vi "Save data file (pass-fail) & report v1.vi"(8 "Input Cluster":T1, 11 "panel id":string) -> (0 "network file save error":errorcluster, 3 "file save path":string)   [LabVIEW 2013]
uses:
  program files/Global 1.vi
  program files/Global display 2.vi
  program files/Global display 3.vi
  <vilib>/Utility/NIReport.llb/NI_report.lvclass
panel:
  out "status":string
  out "C drive root path":string
  out "network file dir path":path
  out "network dir":string
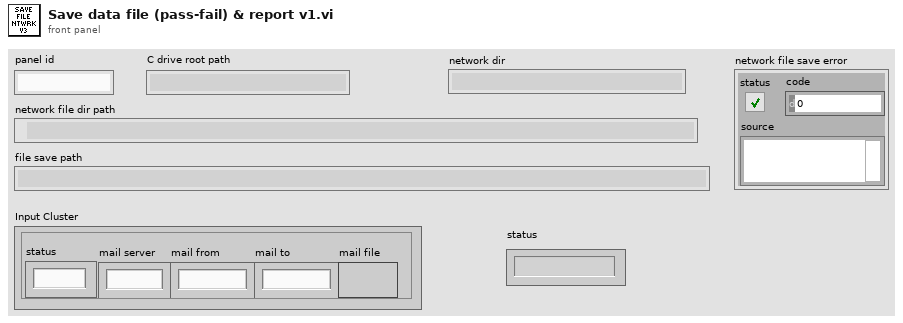
[diagram p1: front panel]
types:
  T1 = cluster{"status":string, "mail server":string, "mail from":string, "mail to":string, "mail file":bool}
  T2 = cluster{"CYCLE":dbl, "MINS":dbl, "STATUS":string}
  T3 = cluster{"NAME":string, "DESCRIPTION":string, "CYCLES":dbl, "T-RISE mins":dbl, "T-RISE deg C":dbl}
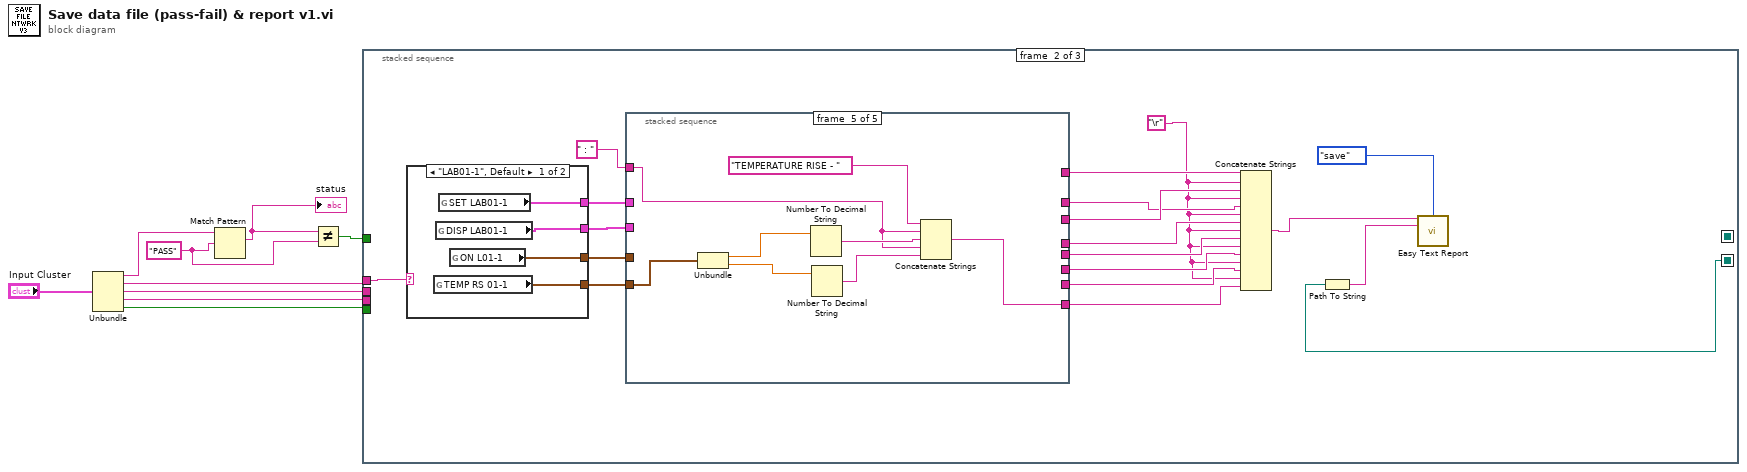
[diagram p0: block diagram]
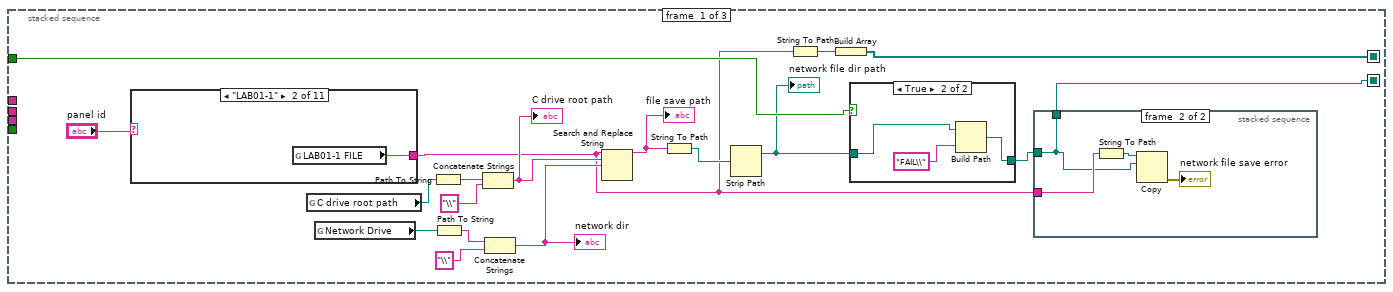
[diagram p2: hidden frame]
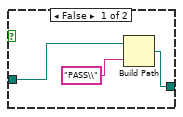
[diagram p3: hidden frame]
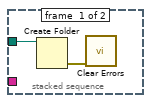
[diagram p4: hidden frame]
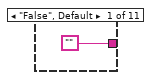
[diagram p5: hidden frame]
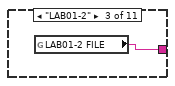
[diagram p6: hidden frame]
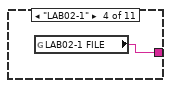
[diagram p7: hidden frame]
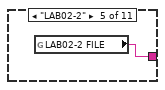
[diagram p8: hidden frame]
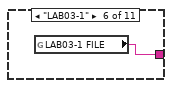
[diagram p9: hidden frame]
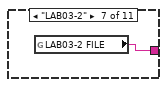
[diagram p10: hidden frame]
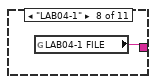
[diagram p11: hidden frame]
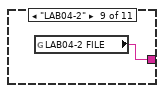
[diagram p12: hidden frame]
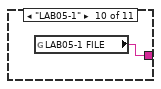
[diagram p13: hidden frame]
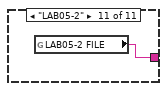
[diagram p14: hidden frame]
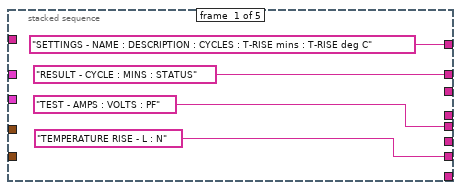
[diagram p15: hidden frame]
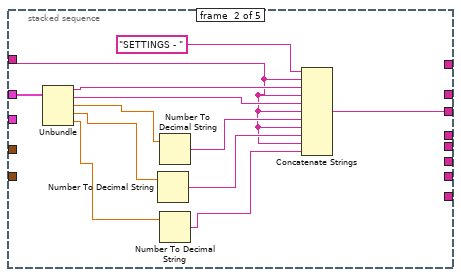
[diagram p16: hidden frame]
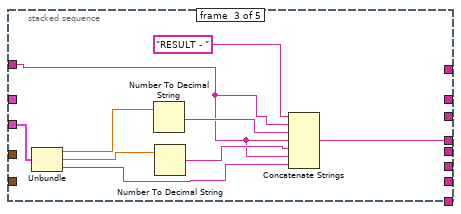
[diagram p17: hidden frame]
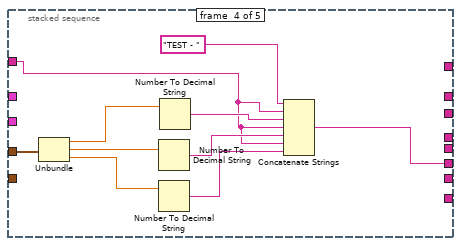
[diagram p18: hidden frame]
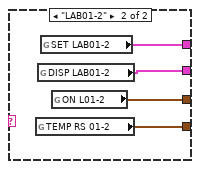
[diagram p19: hidden frame]
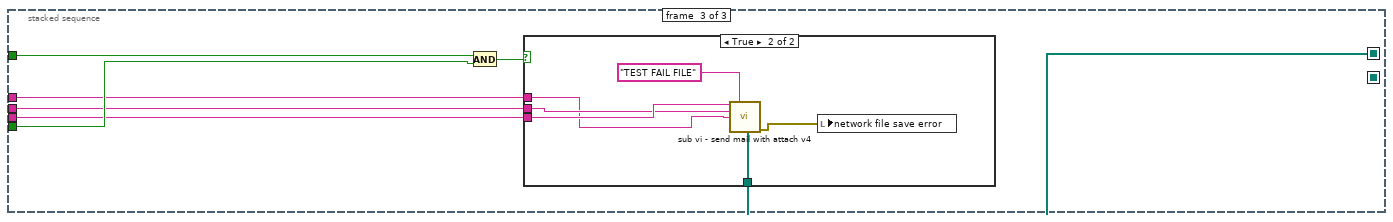
[diagram p20: hidden frame]
diagram:
  w9 = "PASS"
  n1 = Unbundle("Input Cluster") -> ("status"=w7:string, "mail server"=w1:string, "mail from"=w2:string, "mail to"=w3:string, "mail file"=w4:bool)
  n2 = Match Pattern(string=w7, regular expression=w9) -> (match substring=w8:string)  [unwired: 1 in, 3 out]
  "status" <- w8
  n3 = Not Equal?(x=w8, y=w9) -> (x != y?=w5:bool)
  n4 = stacked-sequence {
    seq-local: [w16 _ _] -> [_ _ w126]
    seq-local: [w10 _ _] -> [_ w52 _]
    tunnel: w5 -> [w15 _ w125]
    tunnel: w4 -> [_ _ w124]
    tunnel: w3 -> [_ _ w123]
    tunnel: w2 -> [_ _ w122]
    tunnel: w1 -> [_ w69 w121]
    frame #0 {
      n5 = case shown="\"LAB01-1\"" "panel id" {
        tunnel: ["" w41 w42 w43 w44 w45 w46 w47 w48 w49 w50] -> w11
        frame "False", Default {
        }
        frame "LAB01-1" {
          n6 = global read "Global 1.vi" "LAB01-1 FILE"() -> (w41:string)
        }
        frame "LAB01-2" {
          n7 = global read "Global 1.vi" "LAB01-2 FILE"() -> (w42:string)
        }
        frame "LAB02-1" {
          n8 = global read "Global 1.vi" "LAB02-1 FILE"() -> (w43:string)
        }
        frame "LAB02-2" {
          n9 = global read "Global 1.vi" "LAB02-2 FILE"() -> (w44:string)
        }
        frame "LAB03-1" {
          n10 = global read "Global 1.vi" "LAB03-1 FILE"() -> (w45:string)
        }
        frame "LAB03-2" {
          n11 = global read "Global 1.vi" "LAB03-2 FILE"() -> (w46:string)
        }
        frame "LAB04-1" {
          n12 = global read "Global 1.vi" "LAB04-1 FILE"() -> (w47:string)
        }
        frame "LAB04-2" {
          n13 = global read "Global 1.vi" "LAB04-2 FILE"() -> (w48:string)
        }
        frame "LAB05-1" {
          n14 = global read "Global 1.vi" "LAB05-1 FILE"() -> (w49:string)
        }
        frame "LAB05-2" {
          n15 = global read "Global 1.vi" "LAB05-2 FILE"() -> (w50:string)
        }
      }
      n16 = global read "Global 1.vi" "C drive root path"() -> (w19:path)
      n17 = global read "Global 1.vi" "Network Drive"() -> (w26:path)
      n18 = Path To String(path=w19) -> (string=w20:string)
      n19 = Path To String(path=w26) -> (string=w25:string)
      n20 = Concatenate Strings(w20, "\\") -> (w18:string)
      "C drive root path" <- w18
      n21 = Concatenate Strings(w25, "\\") -> (w23:string)
      "network dir" <- w23
      n22 = Search and Replace String(input string=w11, search string=w18, replace string=w23) -> (result string=w22:string)  [unwired: 5 in, 3 out]
      "file save path" <- w22
      n23 = String To Path(string=w22) -> (path=w17:path)
      n24 = Strip Path(path=w17) -> (stripped path=w13:path)  [unwired: 1 out]
      "network file dir path" <- w13
      n25 = String To Path(string=w11) -> (path=w12:path)
      n26 = Build Array(w12) -> (w16:path[])
      n27 = case shown="True" w15 {
        tunnel: [w28 w33] -> w14
        tunnel: w13 -> [w29 w31]
        frame False {
          n28 = Build Path(base path=w29, name or relative path="PASS\\") -> (appended path=w28:path)
        }
        frame True {
          n29 = Build Path(base path=w31, name or relative path="FAIL\\") -> (appended path=w33:path)
        }
      }
      n30 = stacked-sequence {
        tunnel: w14 -> [w35 w36]
        tunnel: w11 -> [_ w37]
        tunnel: [_ w36] -> w10
        frame #0 {
          n31 = Create Folder(path (use dialog)=w35) -> (error out=w34:errorcluster)  [unwired: 2 in, 2 out]
          n32 = call <vilib>:"Clear Errors.vi"("error in (no error)"=w34) -> ()  [unwired: 6 in, 1 out]
        }
        frame #1 {
          n33 = String To Path(string=w37) -> (path=w38:path)
          n34 = Copy(10:w36, 11:w38) -> (0:→"network file save error":errorcluster)  [unwired: 3 in, 2 out]
        }
      }
    }
    frame #1 {
      w56 = "\r"
      n35 = case shown="\"LAB01-1\", Default" w69 {
        tunnel: [w116 w120] -> w68
        tunnel: [w115 w119] -> w67
        tunnel: [w114 w118] -> w65
        tunnel: [w113 w117] -> w64
        frame "LAB01-1", Default {
          n36 = global read "Global display 3.vi" "TEMP RS 01-1"() -> (w113:cluster{"TL":dbl, "TN":dbl})
          n37 = global read "Global display 2.vi" "DISP LAB01-1"() -> (w115:T2)
          n38 = global read "Global display 2.vi" "SET LAB01-1"() -> (w116:T3)
          n39 = global read "Global display 2.vi" "ON L01-1"() -> (w114:cluster{"amps":dbl, "volts":dbl, "pf":dbl})
        }
        frame "LAB01-2" {
          n40 = global read "Global display 3.vi" "TEMP RS 01-2"() -> (w117:cluster{"TL":dbl, "TN":dbl})
          n41 = global read "Global display 2.vi" "DISP LAB01-2"() -> (w119:T2)
          n42 = global read "Global display 2.vi" "SET LAB01-2"() -> (w120:T3)
          n43 = global read "Global display 2.vi" "ON L01-2"() -> (w118:cluster{"amps":dbl, "volts":dbl, "pf":dbl})
        }
      }
      n44 = stacked-sequence {
        tunnel: w68 -> [_ w85 _ _ _]
        tunnel: w67 -> [_ _ w94 _ _]
        tunnel: " : " -> [_ w75 w87 w96 w107]
        tunnel: w65 -> [_ _ _ w104 _]
        tunnel: w64 -> [_ _ _ _ w112]
        tunnel: ["SETTINGS - NAME : DESCRIPTION : CYCLES : T-RISE mins : T-RISE deg C" _ _ _ _] -> w63
        tunnel: [_ w74 _ _ _] -> w62
        tunnel: ["RESULT - CYCLE : MINS : STATUS" _ _ _ _] -> w61
        tunnel: [_ _ w86 _ _] -> w60
        tunnel: ["TEST - AMPS : VOLTS : PF" _ _ _ _] -> w59
        tunnel: [_ _ _ w95 _] -> w58
        tunnel: ["TEMPERATURE RISE - L : N" _ _ _ _] -> w57
        tunnel: [_ _ _ _ w105] -> w55
        frame #0 {
        }
        frame #1 {
          n45 = Unbundle(w85) -> ("NAME"=w81:string, "DESCRIPTION"=w80:string, "CYCLES"=w84:dbl, "T-RISE mins"=w83:dbl, "T-RISE deg C"=w82:dbl)
          n46 = Number To Decimal String(number=w83) -> (decimal integer string=w78:string)  [unwired: 1 in]
          n47 = Number To Decimal String(number=w84) -> (decimal integer string=w79:string)  [unwired: 1 in]
          n48 = Number To Decimal String(number=w82) -> (decimal integer string=w77:string)  [unwired: 1 in]
          n49 = Concatenate Strings("SETTINGS - ", w75, w81, w75, w80, w75, w79, w75, w78, w75, w77) -> (w74:string)
        }
        frame #2 {
          n50 = Unbundle(w94) -> ("CYCLE"=w93:dbl, "MINS"=w92:dbl, "STATUS"=w89:string)
          n51 = Number To Decimal String(number=w93) -> (decimal integer string=w91:string)  [unwired: 1 in]
          n52 = Number To Decimal String(number=w92) -> (decimal integer string=w90:string)  [unwired: 1 in]
          n53 = Concatenate Strings("RESULT - ", w87, w91, w87, w90, w87, w89) -> (w86:string)
        }
        frame #3 {
          n54 = Unbundle(w104) -> ("amps"=w103:dbl, "volts"=w102:dbl, "pf"=w101:dbl)
          n55 = Number To Decimal String(number=w102) -> (decimal integer string=w99:string)  [unwired: 1 in]
          n56 = Number To Decimal String(number=w101) -> (decimal integer string=w98:string)  [unwired: 1 in]
          n57 = Number To Decimal String(number=w103) -> (decimal integer string=w100:string)  [unwired: 1 in]
          n58 = Concatenate Strings("TEST - ", w96, w100, w96, w99, w96, w98) -> (w95:string)
        }
        frame #4 {
          n59 = Unbundle(w112) -> ("TL"=w111:dbl, "TN"=w110:dbl)
          n60 = Number To Decimal String(number=w111) -> (decimal integer string=w109:string)  [unwired: 1 in]
          n61 = Number To Decimal String(number=w110) -> (decimal integer string=w108:string)  [unwired: 1 in]
          n62 = Concatenate Strings("TEMPERATURE RISE - ", w107, w109, w107, w108) -> (w105:string)
        }
      }
      n63 = Concatenate Strings(w63, w56, w62, w56, w61, w56, w60, w56, w59, w56, w58, w56, w57, w56, w55) -> (w54:string)
      n64 = Path To String(path=w52) -> (string=w51:string)
      n65 = call <vilib>:"Easy Text Report.vi"("text to be printed"=w54, "print or save? (Word/Excel/HTML)"=enum16{"print", "save"}."save", "printer name (default) or file path (dialog)"=w51) -> ()  [unwired: 12 in, 1 out]
    }
    frame #2 {
      n66 = And(x=w125, y=w124) -> (x .and. y?=w127:bool)
      n67 = case shown="True" w127 {
        tunnel: w126 -> [_ w132]
        tunnel: w123 -> [_ w130]
        tunnel: w122 -> [_ w129]
        tunnel: w121 -> [_ w128]
        frame False {
        }
        frame True {
          n68 = call "sub vi - send mail with attach v4.vi"("TO:"=w130, "subject"="TEST FAIL FILE", "from"=w129, "out going server"=w128, "Attachements"=w132) -> ("error out"=w133:errorcluster)  [unwired: 10 in]
          n69 = local write "network file save error"(w133) -> ()
        }
      }
    }
  }
